vi "CloseDevice.vi"(8 "error in (no error)":errorcluster, 11 "CAN-NI in":refnum<class "CAN-NI.lvclass">) -> (0 "error out":errorcluster, 3 "CAN-NI out":refnum<class "CAN-NI.lvclass">)   [LabVIEW 2019, in "CAN-NI.lvlib" / "CAN-NI.lvclass"]
uses:
  CAN-NI.lvclass
  CAN-NI.lvclass/CAN-NI.ctl
  TypeDef/ChannelProperty.ctl
  CAN-Interface/TypeDef/Def-Termination.ctl
  CAN-Interface/TypeDef/Def-Transmit Mode.ctl
  CAN-Interface/TypeDef/Def-Protocol.ctl
  CAN-Interface/Class-Interface.lvclass
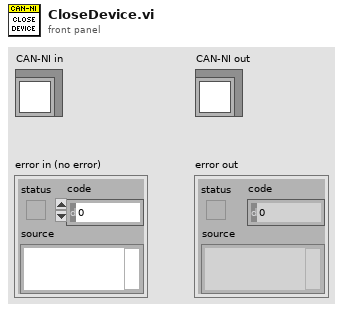
[diagram p1: front panel]
types:
  T1 = typedef "CAN-NI.lvlib/CAN-NI.lvclass/ChannelProperty.ctl" = cluster{"CAN-cluster":refnum<k21>, "CAN-Frames":refnum<k21>[], "Termination":T2, "Transmit Mode":T3, "Frame Out Session":refnum<k21>, "Frame In Session":refnum<k21>, "Protocol":T4}
  T2 = typedef "CAN-Interface.lvlib/Class-Interface.lvclass/Def-Termination.ctl" = enum8{"on", "off"}
  T3 = typedef "CAN-Interface.lvlib/Class-Interface.lvclass/Def-Transmit Mode.ctl" = enum16{"Queued", "Stream"}
  T4 = typedef "CAN-Interface.lvlib/Class-Interface.lvclass/Def-Protocol.ctl" = enum16{"CAN", "CAN FD"}
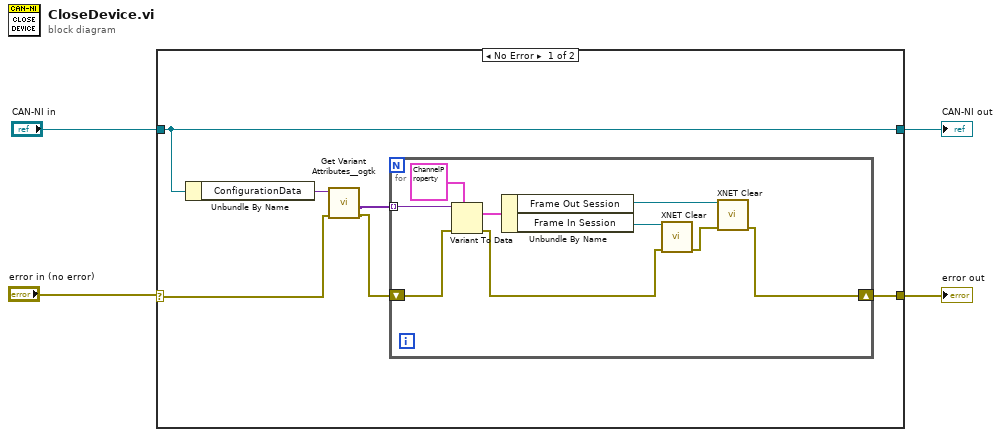
[diagram p0: block diagram]
diagram:
  n1 = case shown="No Error" "error in (no error)" {
    selector: "error in (no error)" -> [w7 w20]
    tunnel: "CAN-NI in" -> [w9 w21]
    tunnel: [w10 w20] -> w2
    tunnel: [w9 w21] -> w1
    frame No Error {
      n2 = Unbundle By Name(w9) -> ("ConfigurationData"=w8:variant)
      n3 = call <userlib>:"Get Variant Attributes__ogtk.vi"("error in"=w7, "Variant"=w8) -> ("error out"=w5:errorcluster, "value(s)"=w6:variant[])  [unwired: 2 in, 2 out]
      n4 = for {
        tunnel: w6 -> [w19] mode=indexing
        shift-right: [w11] -> w10
        shift-left: w5 -> [w18]
        n5 = Variant To Data(error in=w18, type=T1 {"CAN-cluster"="", "CAN-Frames"=[], "Termination"=enum."on", "Transmit Mode"=enum."Queued", "Frame Out Session"="", "Frame In Session"="", "Protocol"=enum."CAN"} ("ChannelProperty"), Variant=w19) -> (data=w16:T1, error out=w13:errorcluster)
        n6 = Unbundle By Name(w16) -> ("Frame Out Session"=w14:refnum<k21>, "Frame In Session"=w15:refnum<k21>)
        n7 = call <vilib>:"XNET Clear.vi"("session in"=w15, "error in (no error)"=w13) -> ("error out"=w12:errorcluster)  [unwired: 13 in]
        n8 = call <vilib>:"XNET Clear.vi"("session in"=w14, "error in (no error)"=w12) -> ("error out"=w11:errorcluster)  [unwired: 13 in]
      }
    }
    frame Error {
    }
  }
  "error out" <- w2
  "CAN-NI out" <- w1
